vi "StateDrivebase.vi"(0 "Master State In":T1(ring)) -> ()   [LabVIEW 2023]
doc: "This VI performs all of the calculations and decisions related to the swerve drive."
uses:
  GlobalDriverStationCommands.vi
  GlobalDriverStationData.vi
  GlobalDrivebase.vi
  GlobalPoseAndTargeting.vi
panel:
  out "Plotting Error":dbl
  out "Current X Strafe Error (in)":dbl
  out "Current Y Strafe Error (in)":dbl
  in  "Strafe PID":T2={"Kp"=0.025, "Ki"=0.0, "Kd"=0.0002, "N-Diff"=10, "N-Int"=20, "Int Error Window"=10.0, "Max Ouput"=0.2, "Min Output"=-0.2, "Square Derivative"=FALSE, "N-Prop"=1} {"N-Prop" min=1; "Int Error Window" min=0.0; "N-Int" min=2; "N-Diff" min=2; "Kd" min=0.0; "Ki" min=0.0; "Kp" min=0.0}
  in  "Plot PID":enum16{"No Plot", "Heading", "Strafe"}(ring)
  out "Strafe Assist On":bool
  in  "Heading Angle PID":T2={"Kp"=0.004, "Ki"=0.0010000000000000002, "Kd"=0.0002, "N-Diff"=10, "N-Int"=10, "Int Error Window"=30.0, "Max Ouput"=1.0, "Min Output"=-1.0, "Square Derivative"=FALSE, "N-Prop"=1} {"N-Prop" min=1; "Int Error Window" min=0.0; "N-Int" min=2; "N-Diff" min=2; "Kd" min=0.0; "Ki" min=0.0; "Kp" min=0.0}
  in  "Acceleration Speed Threshold (ft/s)":dbl=5.0 format="%#_13g"
  out "Module 3 Velocity Command (ul)":dbl(slide) scale=0.0..1.0 scale format="%.2f"
  out "Module 3 Angle (deg)":dbl(knob) scale=180.0..-180.0 scale format="%#_6f"
  out "Module 2 Velocity Command (ul)":dbl(slide) scale=0.0..1.0 scale format="%.2f"
  out "Module 2 Angle (deg)":dbl(knob) scale=180.0..-180.0 scale format="%#_6f"
  out "Module 1 Velocity Command (ul)":dbl(slide) scale=0.0..1.0 scale format="%.2f"
  out "Module 1 Angle (deg)":dbl(knob) scale=180.0..-180.0 scale format="%#_6f"
  out "Module 0 Velocity Command (ul)":dbl(slide) scale=0.0..1.0 scale format="%.2f"
  out "Module 0 Angle (deg)":dbl(knob) scale=180.0..-180.0 scale format="%#_6f"
  in  "Acceleration Limit (ft/s^2)":dbl=80.0
  in  "Speed Cap Decceleration Limit (ft/s^2)":dbl=200.0
  in  "Anti-Drift PID":T2={"Kp"=0.0007, "Ki"=0.0, "Kd"=0.0, "N-Diff"=3, "N-Int"=10, "Int Error Window"=90.0, "Max Ouput"=1.0, "Min Output"=-1.0, "Square Derivative"=FALSE, "N-Prop"=3} {"N-Prop" min=1; "Int Error Window" min=0.0; "N-Int" min=2; "N-Diff" min=2; "Kd" min=0.0; "Ki" min=0.0; "Kp" min=0.0}
  in  "Deceleration Hysteresis (ms)":u32=250
  out "Heading Assist On":bool
  out "PID Plots":T3(graph)
  in  "Heading Fudge Max (deg)":dbl=5.0
  # "\"Front\" of Robot"
  # "M1"
  # "M0"
  # "X"
  # "Y"
  # "(0,0)"
  # "+CCW"
  # "M2"
  # "M3"
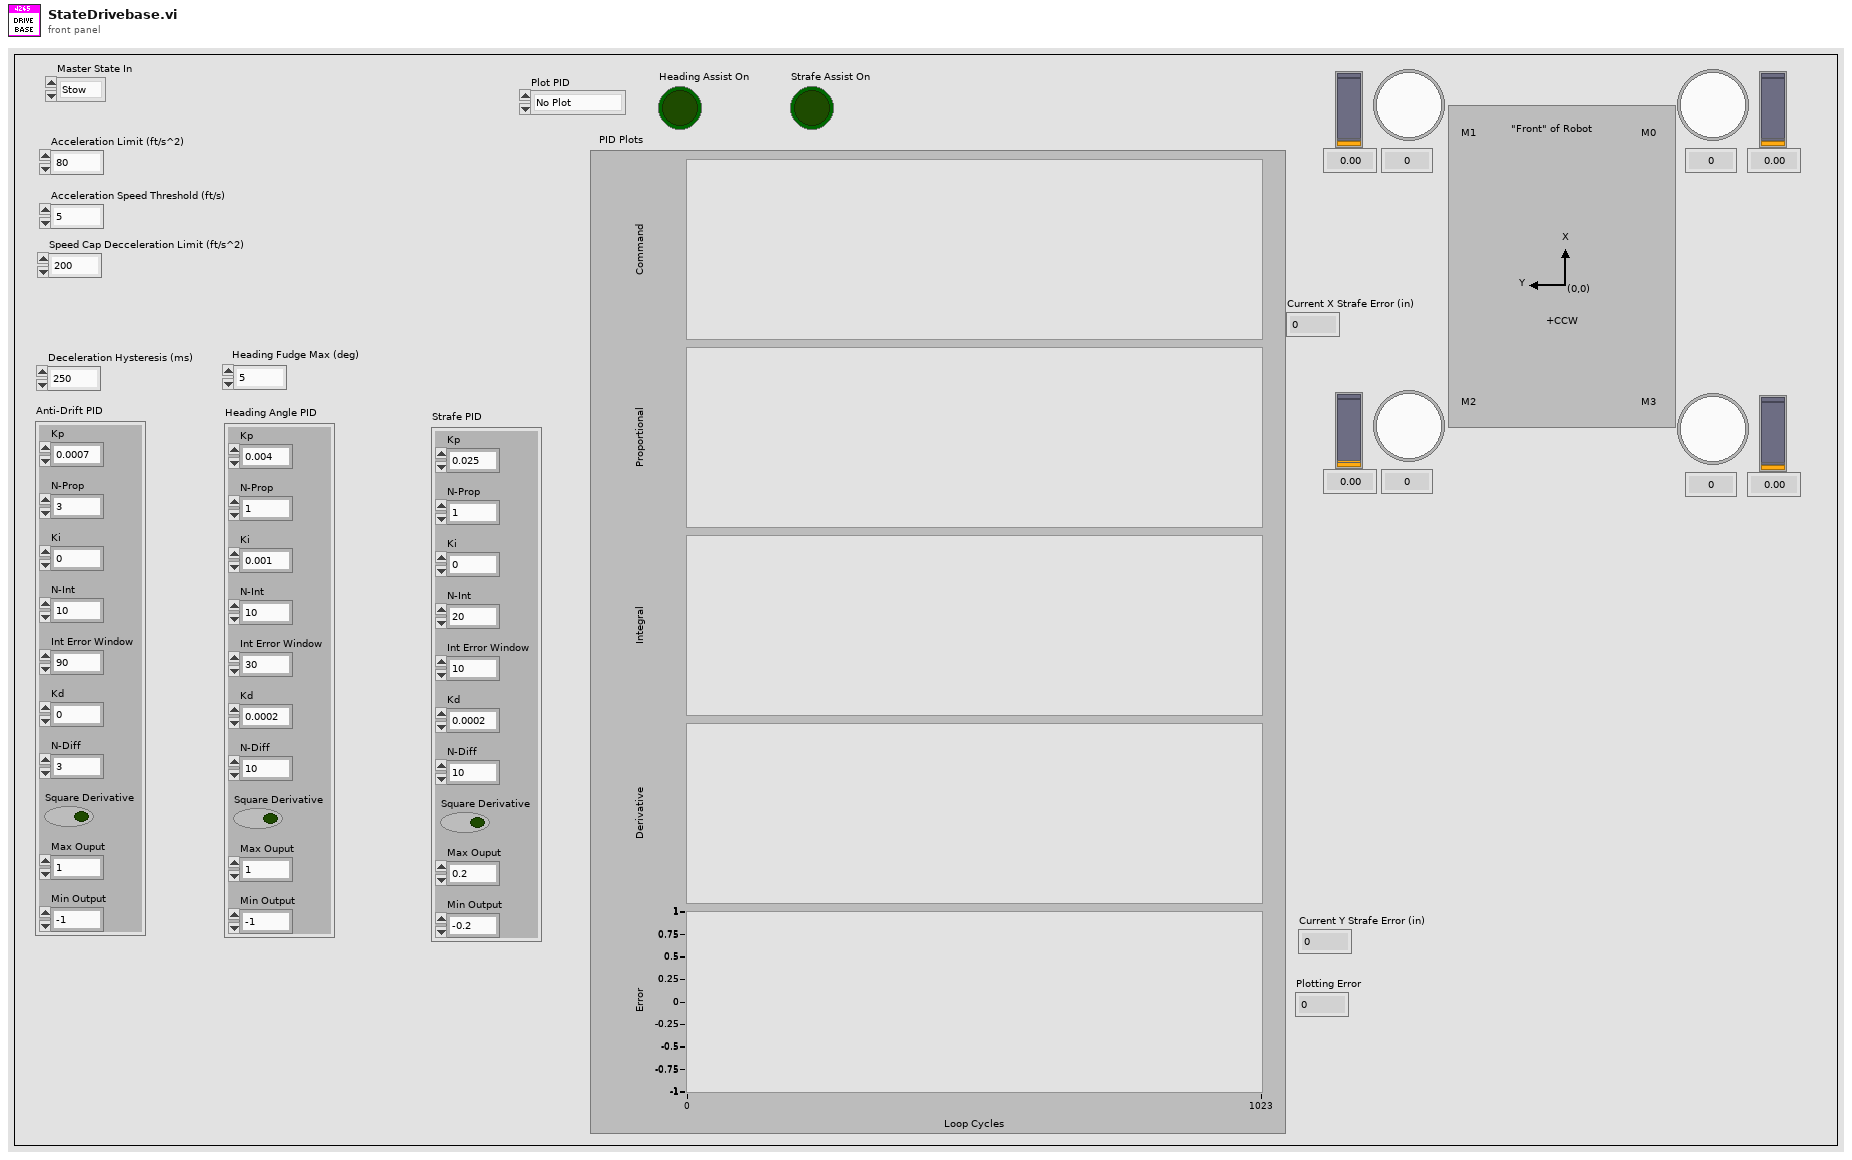
[diagram p1: front panel]
types:
  T1 = enum16{"Stow", "Speaker", "Amp", "Climbing", "Trap"}
  T2 = cluster{"Kp":dbl, "Ki":dbl, "Kd":dbl, "N-Diff":i32, "N-Int":i32, "Int Error Window":dbl, "Max Ouput":dbl, "Min Output":dbl, "Square Derivative":bool, "N-Prop":i32}
  T3 = cluster{"Command":dbl, "Proportional":dbl, "Integral":dbl, "Derivative":dbl, "Goal":dbl}
  T4 = cluster{"Current Setpoints[0]":dbl, "Current Setpoints[1]":dbl, "Current Setpoints[2]":dbl, "Current Setpoints[3]":dbl, "Current Setpoints[4]":dbl, "Current Setpoints[5]":dbl, "Current Setpoints[6]":dbl, "Current Setpoints[7]":dbl, "Current Setpoints[8]":dbl}
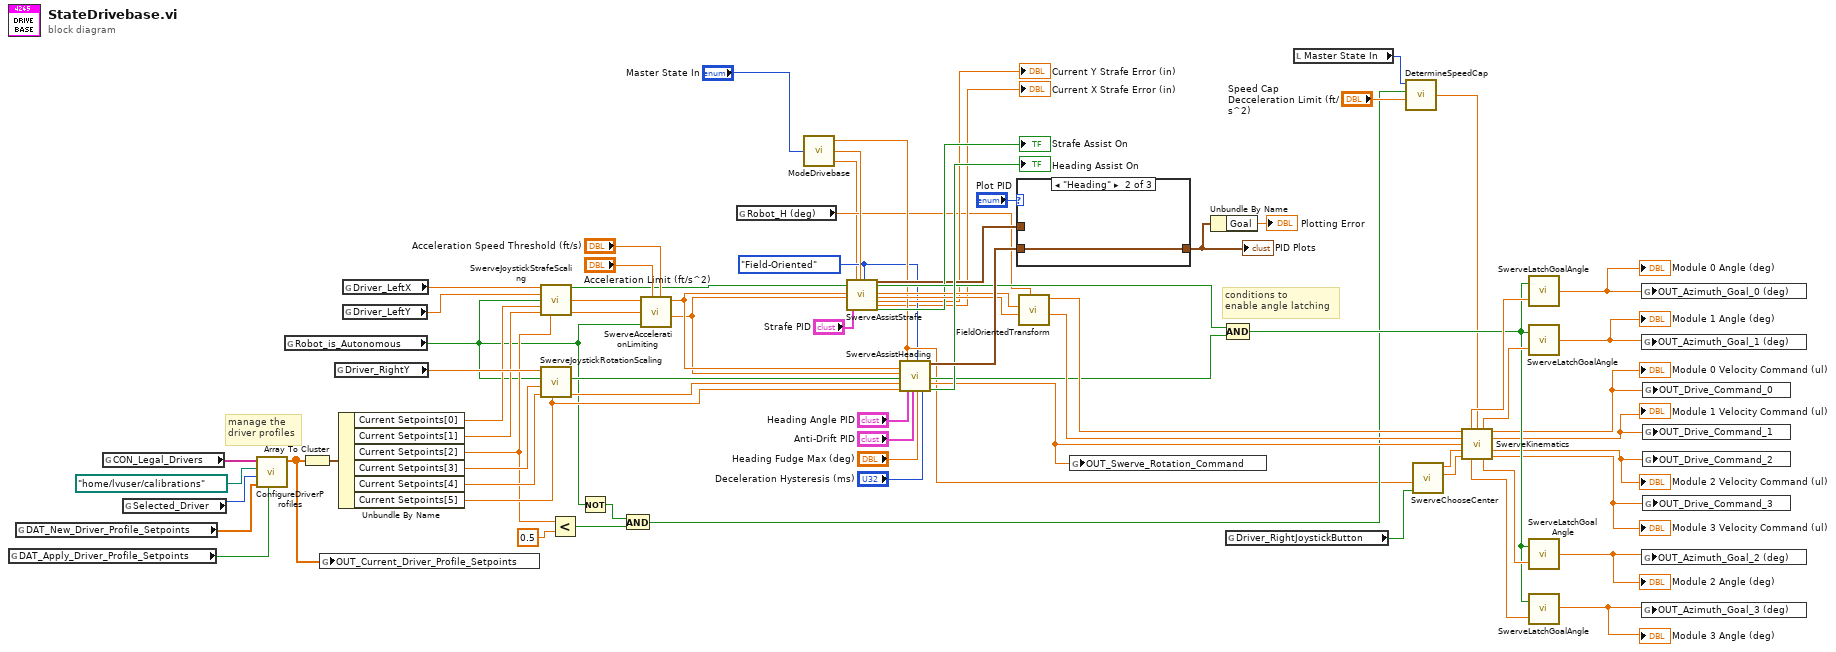
[diagram p0: block diagram]
diagram:
  w8 = enum16{"Robot-Oriented", "Field-Oriented"}."Field-Oriented" ("Orientation Mode")
  # "conditions to\nenable angle latching"
  # "manage the\ndriver profiles"
  n1 = global read "GlobalDrivebase.vi" "DAT_Apply_Driver_Profile_Setpoints"() -> (w50:bool)
  n2 = global read "GlobalDrivebase.vi" "DAT_New_Driver_Profile_Setpoints"() -> (w51:dbl[])
  n3 = global read "GlobalDrivebase.vi" "CON_Legal_Drivers"() -> (w49:string[])
  n4 = global read "GlobalDriverStationData.vi" "Selected_Driver"() -> (w56:i32)
  n5 = call "ConfigureDriverProfiles.vi"("Apply New Setpoint"=w50, "New Setpoints"=w51, "Selected Driver"=w56, "Setpoint Save Location"=path "/home/lvuser/calibrations", "Driver Profile Names"=w49) -> ("Current Setpoints"=w47:dbl[])  [unwired: 6 in]
  n6 = global read "GlobalDriverStationData.vi" "Robot_is_Autonomous"() -> (w11:bool)
  n7 = Array To Cluster(array=w47) -> (cluster=w55:T4)
  n8 = global write "GlobalDrivebase.vi" "OUT_Current_Driver_Profile_Setpoints"(w47) -> ()
  n9 = global read "GlobalDriverStationCommands.vi" "Driver_RightY"() -> (w67:dbl)
  n10 = Unbundle By Name(w55) -> ("Current Setpoints[0]"=w63:dbl, "Current Setpoints[1]"=w62:dbl, "Current Setpoints[2]"=w17:dbl, "Current Setpoints[3]"=w61:dbl, "Current Setpoints[4]"=w60:dbl, "Current Setpoints[5]"=w33:dbl)
  n11 = global read "GlobalDriverStationCommands.vi" "Driver_LeftX"() -> (w70:dbl)
  n12 = global read "GlobalDriverStationCommands.vi" "Driver_LeftY"() -> (w69:dbl)
  n13 = call "SwerveJoystickStrafeScaling.vi"("Raw Joystick X"=w70, "Raw Joystick Y"=w69, "Auto Control"=w11, "Strafe Deadband"=w63, "Strafe Scaling"=w62, "Strafe Maximum"=w17) -> ("In Deadband"=w23:bool, "Scaled Joystick X"=w45:dbl, "Scaled Joystick Y"=w44:dbl)  [unwired: 7 in]
  n14 = call "SwerveJoystickRotationScaling.vi"("Rotation Maximum"=w33, "Rotation Scaling"=w60, "Rotation Deadband"=w61, "Auto Control"=w11, "Raw Joystick Rotation"=w67) -> ("Scaled Joystick Rotation"=w68:dbl, "In Deadband"=w32:bool)  [unwired: 4 in]
  n15 = Less?(x=w17, y=0.5) -> (x < y?=w30:bool)
  n16 = Not(x=w11) -> (.not. x?=w28:bool)
  n17 = And(x=w28, y=w30) -> (x .and. y?=w29:bool)
  n18 = call "SwerveAccelerationLimiting.vi"("Min Speed Threshold (ft/s)"="Acceleration Speed Threshold (ft/s)", "Acceleration Limit (ft/s^2)"="Acceleration Limit (ft/s^2)", "Auto Control"=w11, "Joystick Y"=w44, "Joystick X"=w45) -> ("Limited Joystick Y"=w20:dbl, "Limited Joystick X"=w21:dbl)  [unwired: 5 in]
  n19 = global read "GlobalPoseAndTargeting.vi" "Robot_H (deg)"() -> (w5:dbl)
  n20 = call "ModeDrivebase.vi"("Master State In"="Master State In") -> ("Locked Heading (deg)"=w10:dbl, "Locked Y (in)"=w13:dbl, "Locked X (in)"=w4:dbl)
  n21 = call "SwerveAssistStrafe.vi"("In Deadband"=w23, "Joystick X"=w21, "Joystick Y"=w20, "Strafe PID"="Strafe PID", "Locked X (in)"=w4, "Locked Y (in)"=w13, "Orientation Mode"=w8) -> ("Strafe PID Plot"=w15:T3, "In Deadband"=w22:bool, "Assisted X"=w18:dbl, "Assisted Y"=w19:dbl, "Current Y Error (in)"=→"Current Y Strafe Error (in)":dbl, "Current X Error (in)"=→"Current X Strafe Error (in)":dbl, "Strafe Assist On"=→"Strafe Assist On":bool)  [unwired: 14 in]
  n22 = call "SwerveAssistHeading.vi"("Joystick X"=w21, "Joystick Y"=w20, "In Deadband"=w32, "Joystick Rotation"=w68, "Rotation Maximum"=w33, "Locked Heading (deg) [0,360]"=w10, "Heading Angle PID"="Heading Angle PID", "Anti-Drift PID"="Anti-Drift PID", "Orientation Mode"=w8, "Heading Fudge Max (deg)"="Heading Fudge Max (deg)", "Deceleration Hysteresis (ms)"="Deceleration Hysteresis (ms)") -> ("Heading PID Plot"=w72:T3, "In Deadband"=w31:bool, "Assisted Rotation"=w48:dbl, "Heading Assist On"=→"Heading Assist On":bool)  [unwired: 5 in]
  n23 = case shown="\"Heading\"" "Plot PID" {
    tunnel: w72 -> [_ w77 _]
    tunnel: w15 -> [_ _ w78]
    tunnel: [_ w77 w78] -> w3
    frame "No Plot", Default {
    }
    frame "Heading" {
    }
    frame "Strafe" {
    }
  }
  "PID Plots" <- w3
  n24 = call "FieldOrientedTransform.vi"("Robot Oriented Direction (deg)"=w5, "Joystick Y"=w19, "Joystick X"=w18) -> ("Joystick Y'"=w64:dbl, "Joystick X'"=w66:dbl)  [unwired: 7 in]
  n25 = global write "GlobalDrivebase.vi" "OUT_Swerve_Rotation_Command"(w48) -> ()
  n26 = Unbundle By Name(w3) -> ("Goal"=→"Plotting Error":dbl)
  n27 = global read "GlobalDriverStationCommands.vi" "Driver_RightJoystickButton"() -> (w71:bool)
  n28 = Compound Arithmetic op=AND(w22, w31) -> (w53:bool)
  n29 = local read "Master State In"() -> (w1:T1)
  n30 = call "DetermineSpeedCap.vi"("Speed Cap Decceleration Limit (ft/s^2)"="Speed Cap Decceleration Limit (ft/s^2)", "Driver Profile Doesn't Want to Shift"=w29, "Master State In"=w1) -> ("Speed Cap [0,1]"=w52:dbl)  [unwired: 1 in]
  n31 = call "SwerveChooseCenter.vi"("Corner Pivot Trigger"=w71, "Locked Heading (deg)"=w10) -> ("Cy (in)"=w58:dbl, "Cx (in)"=w59:dbl)  [unwired: 6 in]
  n32 = call "SwerveKinematics.vi"("Joystick X"=w66, "Saturation Velocity (ul)"=w52, "Joystick Y"=w64, "Joystick Rotation"=w48, "Cx (in)"=w59, "Cy (in)"=w58) -> ("Module 0 Angle (deg)"=w76:dbl, "Module 1 Angle (deg)"=w75:dbl, "Module 0 Velocity Command (ul)"=w42:dbl, "Module 1 Velocity Command (ul)"=w41:dbl, "Module 2 Velocity Command (ul)"=w40:dbl, "Module 3 Angle (deg)"=w73:dbl, "Module 2 Angle (deg)"=w74:dbl, "Module 3 Velocity Command (ul)"=w39:dbl)  [unwired: 2 in]
  "Module 0 Velocity Command (ul)" <- w42
  "Module 1 Velocity Command (ul)" <- w41
  "Module 2 Velocity Command (ul)" <- w40
  "Module 3 Velocity Command (ul)" <- w39
  n33 = call "SwerveLatchGoalAngle.vi"("Raw Goal Angle"=w76, "In Deadband"=w53) -> ("Latched Goal Angle"=w36:dbl)
  "Module 0 Angle (deg)" <- w36
  n34 = call "SwerveLatchGoalAngle.vi"("Raw Goal Angle"=w75, "In Deadband"=w53) -> ("Latched Goal Angle"=w37:dbl)
  "Module 1 Angle (deg)" <- w37
  n35 = call "SwerveLatchGoalAngle.vi"("Raw Goal Angle"=w74, "In Deadband"=w53) -> ("Latched Goal Angle"=w38:dbl)
  "Module 2 Angle (deg)" <- w38
  n36 = call "SwerveLatchGoalAngle.vi"("Raw Goal Angle"=w73, "In Deadband"=w53) -> ("Latched Goal Angle"=w35:dbl)
  "Module 3 Angle (deg)" <- w35
  n37 = global write "GlobalDrivebase.vi" "OUT_Azimuth_Goal_0 (deg)"(w36) -> ()
  n38 = global write "GlobalDrivebase.vi" "OUT_Azimuth_Goal_1 (deg)"(w37) -> ()
  n39 = global write "GlobalDrivebase.vi" "OUT_Azimuth_Goal_2 (deg)"(w38) -> ()
  n40 = global write "GlobalDrivebase.vi" "OUT_Azimuth_Goal_3 (deg)"(w35) -> ()
  n41 = global write "GlobalDrivebase.vi" "OUT_Drive_Command_0"(w42) -> ()
  n42 = global write "GlobalDrivebase.vi" "OUT_Drive_Command_1"(w41) -> ()
  n43 = global write "GlobalDrivebase.vi" "OUT_Drive_Command_2"(w40) -> ()
  n44 = global write "GlobalDrivebase.vi" "OUT_Drive_Command_3"(w39) -> ()
